vi "Close_RFSAP2P.vi"(0 "reference":refnum<vi>, 5 "Control Name":string="clear err", 7 "Boolean":bool=TRUE) -> (15 "error out":errorcluster)   [LabVIEW 2019]
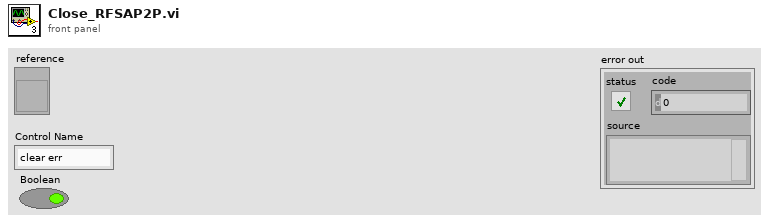
[diagram p1: front panel]
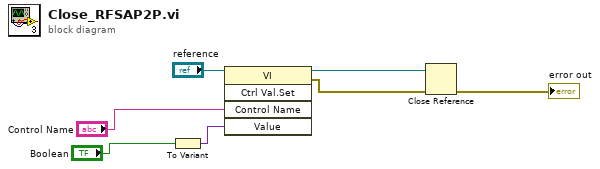
[diagram p0: block diagram]
diagram:
  n1 = To Variant(anything="Boolean") -> (Variant=w4:variant)
  n2 = invoke class="VI" method="Ctrl Val.Set"(reference="reference", "Control Name"="Control Name", "Value"=w4) -> (reference out=w1:refnum<vi>, error out=w7:errorcluster)  [unwired: 2 in, 3 out]
  n3 = Close Reference(reference=w1, error in (no error)=w7) -> (error out=→"error out":errorcluster)
